vi "WILT Station Controller.vi"(0 "Station Number":u32, 1 "GUI Aisle in":T9[](array[typedef]) {"Night Cycle Count" format="%04d"; "Day Cycle Count" format="%04d"}, 3 "Drying Time (Min)":dbl[](array[numeric]), 4 "Current Threshold":dbl=1.0 format="%#_13g", 5 "Station Test State In":T7, 7 "Error In":errorcluster, 8 "Aisle Location Index":i32, 9 "Cool Down Period (seconds)":dbl[](array[numeric]), 10 "Disable Flood Check":bool, 11 "Delay After Cutout (sec)":dbl=5.0 format="%#_13g", 12 "Previous Run Statistics":T2[](array[typedef]), 13 "Send Restart Every? (Sec)":dbl=7.0 format="%#_13g", 14 "Agilent Valve and Switch Locations":T3[](array[typedef])=[{"Channel"="301", "Station"="1", "Label"="Water Valve", "Agilent Station"="2", "Data"=0.0}, {"Channel"="302", "Station"="2", "Label"="Water Valve", "Agilent Station"="2", "Data"=0.0}, {"Channel"="303", "Station"="3", "Label"="Water Valve", "Agilent Station"="2", "Data"=0.0}, {"Channel"="304", "Station"="4", "Label"="Water Valve", "Agilent Station"="2", "Data"=0.0}, {"Channel"="305", "Station"="5", "Label"="Water Valve", "Agilent Station"="2", "Data"=0.0}, {"Channel"="306", "Station"="6", "Label"="Water Valve", "Agilent Station"="2", "Data"=0.0}, {"Channel"="307", "Station"="7", "Label"="Water Valve", "Agilent Station"="2", "Data"=0.0}, {"Channel"="308", "Station"="8", "Label"="Water Valve", "Agilent Station"="2", "Data"=0.0}, {"Channel"="309", "Station"="9", "Label"="Water Valve", "Agilent Station"="2", "Data"=0.0}, {"Channel"="310", "Station"="10", "Label"="Water Valve", "Agilent Station"="2", "Data"=0.0}, {"Channel"="311", "Station"="11", "Label"="Water Valve", "Agilent Station"="2", "Data"=0.0}, {"Channel"="312", "Station"="12", "Label"="Water Valve", "Agilent Station"="2", "Data"=0.0}, {"Channel"="313", "Station"="13", "Label"="Water Valve", "Agilent Station"="2", "Data"=0.0}, {"Channel"="314", "Station"="14", "Label"="Water Valve", "Agilent Station"="2", "Data"=0.0}, {"Channel"="315", "Station"="15", "Label"="Water Valve", "Agilent Station"="2", "Data"=0.0}, {"Channel"="316", "Station"="16", "Label"="Water Valve", "Agilent Station"="2", "Data"=0.0}, {"Channel"="317", "Station"="17", "Label"="Water Valve", "Agilent Station"="2", "Data"=0.0}, {"Channel"="318", "Station"="18", "Label"="Water Valve", "Agilent Station"="2", "Data"=0.0}, {"Channel"="319", "Station"="19", "Label"="Water Valve", "Agilent Station"="2", "Data"=0.0}, {"Channel"="320", "Station"="20", "Label"="Water Valve", "Agilent Station"="2", "Data"=0.0}, {"Channel"="101", "Station"="21", "Label"="Water Valve", "Agilent Station"="3", "Data"=0.0}, {"Channel"="102", "Station"="22", "Label"="Water Valve", "Agilent Station"="3", "Data"=0.0}, {"Channel"="103", "Station"="23", "Label"="Water Valve", "Agilent Station"="3", "Data"=0.0}, {"Channel"="104", "Station"="24", "Label"="Water Valve", "Agilent Station"="3", "Data"=0.0}, {"Channel"="105", "Station"="25", "Label"="Water Valve", "Agilent Station"="3", "Data"=0.0}, {"Channel"="106", "Station"="26", "Label"="Water Valve", "Agilent Station"="3", "Data"=0.0}, {"Channel"="107", "Station"="27", "Label"="Water Valve", "Agilent Station"="3", "Data"=0.0}, {"Channel"="108", "Station"="28", "Label"="Water Valve", "Agilent Station"="3", "Data"=0.0}, {"Channel"="109", "Station"="29", "Label"="Water Valve", "Agilent Station"="3", "Data"=0.0}, {"Channel"="110", "Station"="30", "Label"="Water Valve", "Agilent Station"="3", "Data"=0.0}, {"Channel"="111", "Station"="31", "Label"="Water Valve", "Agilent Station"="3", "Data"=0.0}, {"Channel"="112", "Station"="32", "Label"="Water Valve", "Agilent Station"="3", "Data"=0.0}, {"Channel"="101", "Station"="33", "Label"="Water Valve", "Agilent Station"="5", "Data"=0.0}, {"Channel"="102", "Station"="34", "Label"="Water Valve", "Agilent Station"="5", "Data"=0.0}, {"Channel"="103", "Station"="35", "Label"="Water Valve", "Agilent Station"="5", "Data"=0.0}, {"Channel"="104", "Station"="36", "Label"="Water Valve", "Agilent Station"="5", "Data"=0.0}, {"Channel"="105", "Station"="37", "Label"="Water Valve", "Agilent Station"="5", "Data"=0.0}, {"Channel"="106", "Station"="38", "Label"="Water Valve", "Agilent Station"="5", "Data"=0.0}, {"Channel"="107", "Station"="39", "Label"="Water Valve", "Agilent Station"="5", "Data"=0.0}, {"Channel"="108", "Station"="40", "Label"="Water Valve", "Agilent Station"="5", "Data"=0.0}, {"Channel"="109", "Station"="41", "Label"="Water Valve", "Agilent Station"="5", "Data"=0.0}, {"Channel"="110", "Station"="42", "Label"="Water Valve", "Agilent Station"="5", "Data"=0.0}, {"Channel"="111", "Station"="43", "Label"="Water Valve", "Agilent Station"="5", "Data"=0.0}, {"Channel"="112", "Station"="44", "Label"="Water Valve", "Agilent Station"="5", "Data"=0.0}, {"Channel"="113", "Station"="45", "Label"="Water Valve", "Agilent Station"="5", "Data"=0.0}, {"Channel"="114", "Station"="46", "Label"="Water Valve", "Agilent Station"="5", "Data"=0.0}, {"Channel"="115", "Station"="47", "Label"="Water Valve", "Agilent Station"="5", "Data"=0.0}, {"Channel"="116", "Station"="48", "Label"="Water Valve", "Agilent Station"="5", "Data"=0.0}, {"Channel"="117", "Station"="49", "Label"="Water Valve", "Agilent Station"="5", "Data"=0.0}, {"Channel"="118", "Station"="50", "Label"="Water Valve", "Agilent Station"="5", "Data"=0.0}, {"Channel"="119", "Station"="51", "Label"="Water Valve", "Agilent Station"="5", "Data"=0.0}, {"Channel"="120", "Station"="52", "Label"="Water Valve", "Agilent Station"="5", "Data"=0.0}, {"Channel"="201", "Station"="53", "Label"="Water Valve", "Agilent Station"="5", "Data"=0.0}, {"Channel"="202", "Station"="54", "Label"="Water Valve", "Agilent Station"="5", "Data"=0.0}, {"Channel"="203", "Station"="55", "Label"="Water Valve", "Agilent Station"="5", "Data"=0.0}, {"Channel"="204", "Station"="56", "Label"="Water Valve", "Agilent Station"="5", "Data"=0.0}, {"Channel"="301", "Station"="21", "Label"="Start Button", "Agilent Station"="5", "Data"=0.0}, {"Channel"="302", "Station"="22", "Label"="Start Button", "Agilent Station"="5", "Data"=0.0}, {"Channel"="303", "Station"="23", "Label"="Start Button", "Agilent Station"="5", "Data"=0.0}, {"Channel"="304", "Station"="24", "Label"="Start Button", "Agilent Station"="5", "Data"=0.0}, {"Channel"="305", "Station"="25", "Label"="Start Button", "Agilent Station"="5", "Data"=0.0}, {"Channel"="306", "Station"="26", "Label"="Start Button", "Agilent Station"="5", "Data"=0.0}, {"Channel"="307", "Station"="27", "Label"="Start Button", "Agilent Station"="5", "Data"=0.0}, {"Channel"="308", "Station"="28", "Label"="Start Button", "Agilent Station"="5", "Data"=0.0}, {"Channel"="309", "Station"="29", "Label"="Start Button", "Agilent Station"="5", "Data"=0.0}, {"Channel"="310", "Station"="30", "Label"="Start Button", "Agilent Station"="5", "Data"=0.0}, {"Channel"="311", "Station"="31", "Label"="Start Button", "Agilent Station"="5", "Data"=0.0}, {"Channel"="312", "Station"="32", "Label"="Start Button", "Agilent Station"="5", "Data"=0.0}, {"Channel"="101", "Station"="33", "Label"="Start Button", "Agilent Station"="7", "Data"=0.0}, {"Channel"="102", "Station"="34", "Label"="Start Button", "Agilent Station"="7", "Data"=0.0}, {"Channel"="103", "Station"="35", "Label"="Start Button", "Agilent Station"="7", "Data"=0.0}, {"Channel"="104", "Station"="36", "Label"="Start Button", "Agilent Station"="7", "Data"=0.0}, {"Channel"="105", "Station"="37", "Label"="Start Button", "Agilent Station"="7", "Data"=0.0}, {"Channel"="106", "Station"="38", "Label"="Start Button", "Agilent Station"="7", "Data"=0.0}, {"Channel"="107", "Station"="39", "Label"="Start Button", "Agilent Station"="7", "Data"=0.0}, {"Channel"="108", "Station"="40", "Label"="Start Button", "Agilent Station"="7", "Data"=0.0}, {"Channel"="109", "Station"="41", "Label"="Start Button", "Agilent Station"="7", "Data"=0.0}, {"Channel"="110", "Station"="42", "Label"="Start Button", "Agilent Station"="7", "Data"=0.0}, {"Channel"="111", "Station"="43", "Label"="Start Button", "Agilent Station"="7", "Data"=0.0}, {"Channel"="112", "Station"="44", "Label"="Start Button", "Agilent Station"="7", "Data"=0.0}, {"Channel"="113", "Station"="45", "Label"="Start Button", "Agilent Station"="7", "Data"=0.0}, {"Channel"="114", "Station"="46", "Label"="Start Button", "Agilent Station"="7", "Data"=0.0}, {"Channel"="115", "Station"="47", "Label"="Start Button", "Agilent Station"="7", "Data"=0.0}, {"Channel"="116", "Station"="48", "Label"="Start Button", "Agilent Station"="7", "Data"=0.0}, {"Channel"="117", "Station"="49", "Label"="Start Button", "Agilent Station"="7", "Data"=0.0}, {"Channel"="118", "Station"="50", "Label"="Start Button", "Agilent Station"="7", "Data"=0.0}, {"Channel"="119", "Station"="51", "Label"="Start Button", "Agilent Station"="7", "Data"=0.0}, {"Channel"="120", "Station"="52", "Label"="Start Button", "Agilent Station"="7", "Data"=0.0}, {"Channel"="201", "Station"="53", "Label"="Start Button", "Agilent Station"="7", "Data"=0.0}, {"Channel"="202", "Station"="54", "Label"="Start Button", "Agilent Station"="7", "Data"=0.0}, {"Channel"="203", "Station"="55", "Label"="Start Button", "Agilent Station"="7", "Data"=0.0}, {"Channel"="204", "Station"="56", "Label"="Start Button", "Agilent Station"="7", "Data"=0.0}], 15 "Injection Times":T4, 16 "Enable Start Retry":bool[](array[boolean]), 17 "Day/Night Cycle":T6, 19 "Final Start Presses":i32=2, 25 "Semaphore":T1[](array[typedef])) -> (20 "GUI Aisle 1":T9[](array[typedef]) {"Night Cycle Count" format="%04d"; "Day Cycle Count" format="%04d"}, 21 "Test Station Out":T7, 23 "Resending Sending Command":bool, 24 "Enable Start Retry Out":bool[](array[boolean]), 27 "Error Out":errorcluster)   [LabVIEW 2016]
uses:
  Type Definitions/WILT Dryer.ctl
  Type Definitions/WILT Dryer Details.ctl
  Type Definitions/WILT Agilent Channel Definition.ctl
  Type Definitions/WILT DAQ Data.ctl
  Type Definitions/WILT Station Test State Cluster.ctl
  Type Definitions/WILT Dryer Test State.ctl
  Type Definitions/WILT Day Night Cycle Enum.ctl
  Type Definitions/WILT Injection Times.ctl
  Type Definitions/WILT Water Injection Control.ctl
  Type Definitions/WILT Summary Data.ctl
  Type Definitions/WILT Water Valve Control.ctl
  Type Definitions/WILT Room Location.ctl
panel:
  out "56":dbl
  out "55":dbl
  out "54":dbl
  out "53":dbl
  out "52":dbl
  out "51":dbl
  out "50":dbl
  out "49":dbl
  out "48":dbl
  out "47":dbl
  out "46":dbl
  out "45":dbl
  out "44":dbl
  out "43":dbl
  out "42":dbl
  out "41":dbl
  out "40":dbl
  out "39":dbl
  out "38":dbl
  out "37":dbl
  out "36":dbl
  out "35":dbl
  out "34":dbl
  out "33":dbl
  out "32":dbl
  out "31":dbl
  out "30":dbl
  out "29":dbl
  out "28":dbl
  out "27":dbl
  out "26":dbl
  out "25":dbl
  out "24":dbl
  out "23":dbl
  out "22":dbl
  out "21":dbl
  out "20":dbl
  out "19":dbl
  out "18":dbl
  out "17":dbl
  out "16":dbl
  out "15":dbl
  out "14":dbl
  out "13":dbl
  out "12":dbl
  out "11":dbl
  out "10":dbl
  out "9":dbl
  out "8":dbl
  out "7":dbl
  out "6":dbl
  out "5":dbl
  out "4":dbl
  out "3":dbl
  out "2":dbl
  out "1":dbl
  # "Individual Station Timers"
  # "Day"
  # "Night"
  # "Day"
  # "Night"
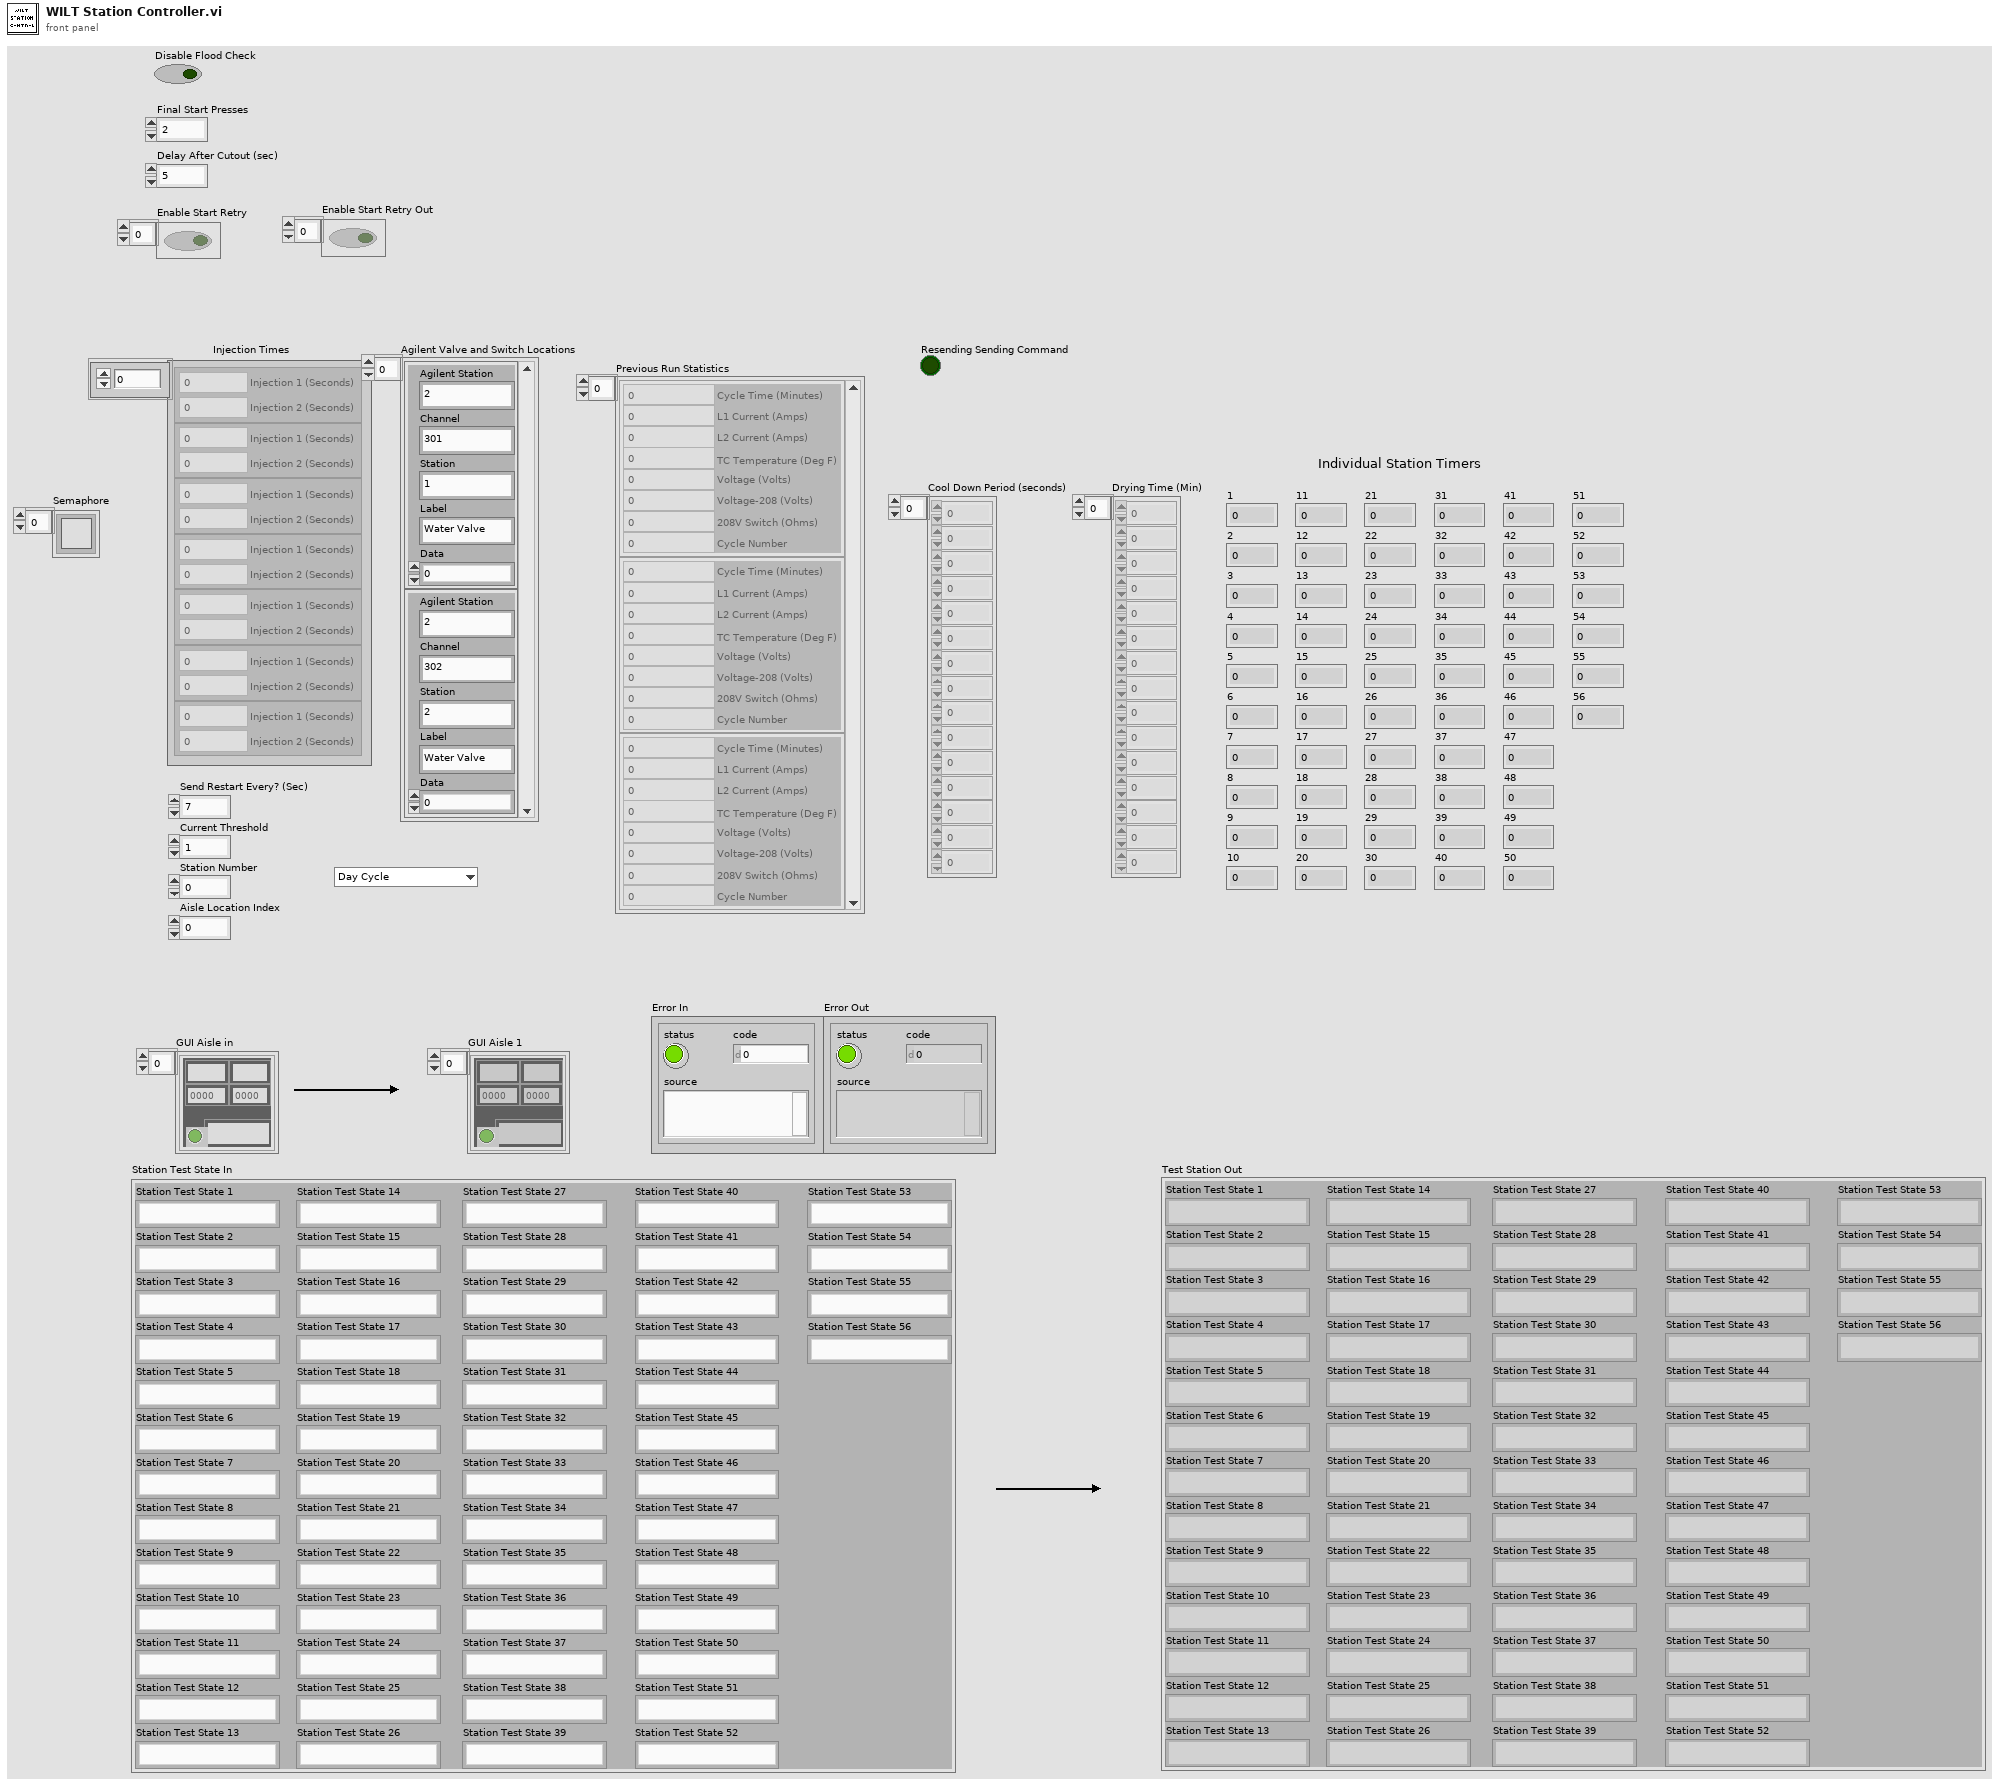
[diagram p1: front panel]
types:
  T1 = typedef "Semaphore RefNum" = refnum<k1>
  T2 = typedef "WILT Summary Data.ctl" = cluster{"Cycle Time (Minutes)":dbl, "L1 Current (Amps)":dbl, "L2 Current (Amps)":dbl, "TC Temperature (Deg F)":dbl, "Voltage (Volts)":dbl, "Voltage-208 (Volts)":dbl, "208V Switch (Ohms)":dbl, "Cycle Number":i32}
  T3 = typedef "WILT Agilent Channel Definition.ctl" = cluster{"Channel":string, "Station":string, "Label":string, "Agilent Station":string, "Data":dbl}
  T4 = typedef "WILT Injection Times.ctl" = T5[]
  T5 = typedef "WILT Water Injection Control.ctl" = cluster{"Injection 1 (Seconds)":dbl, "Injection 2 (Seconds)":dbl}
  T6 = typedef "WILT Day Night Cycle Enum.ctl" = enum16{"Day Cycle", "Night Cycle", "Day Cycle (No Water)"}
  T7 = typedef "WILT Station Test State Cluster.ctl" = cluster{"Station Test State 1":T8, "Station Test State 2":T8, "Station Test State 3":T8, "Station Test State 4":T8, "Station Test State 5":T8, "Station Test State 6":T8, "Station Test State 7":T8, "Station Test State 8":T8, "Station Test State 9":T8, "Station Test State 10":T8, "Station Test State 11":T8, "Station Test State 12":T8, "Station Test State 13":T8, "Station Test State 14":T8, "Station Test State 15":T8, "Station Test State 16":T8, "Station Test State 17":T8, "Station Test State 18":T8, "Station Test State 19":T8, "Station Test State 20":T8, "Station Test State 21":T8, "Station Test State 22":T8, "Station Test State 23":T8, "Station Test State 24":T8, "Station Test State 25":T8, "Station Test State 26":T8, "Station Test State 27":T8, "Station Test State 28":T8, "Station Test State 29":T8, "Station Test State 30":T8, "Station Test State 31":T8, "Station Test State 32":T8, "Station Test State 33":T8, "Station Test State 34":T8, "Station Test State 35":T8, "Station Test State 36":T8, "Station Test State 37":T8, "Station Test State 38":T8, "Station Test State 39":T8, "Station Test State 40":T8, "Station Test State 41":T8, "Station Test State 42":T8, "Station Test State 43":T8, "Station Test State 44":T8, "Station Test State 45":T8, "Station Test State 46":T8, "Station Test State 47":T8, "Station Test State 48":T8, "Station Test State 49":T8, "Station Test State 50":T8, "Station Test State 51":T8, "Station Test State 52":T8, "Station Test State 53":T8, "Station Test State 54":T8, "Station Test State 55":T8, "Station Test State 56":T8}
  T8 = typedef "WILT Dryer Test State.ctl" = enum16{"No Serial Number", "Waiting for Dryer To Start", "Drying Clothes", "Water Injection 1 (On)", "Water Injection 1 Timer", "Water Injection 1 (Off)", "Pause Dryer", "Sending Start Stop CMD", "Pause Dryer 2", "Sending Start Stop CMD 2", "Drying Clothes 2", "Water Injection 2 (On)", "Water Injection 2 Timer", "Water Injection 2 (Off)", "Drying Clothes 3", "Cooling Down", "Sending Start Stop CMD 3", "Increment Cycle"}
  T9 = typedef "WILT Dryer.ctl" = cluster{"Lab ID":string, "Day Cycle Count":i32, "Station Label":string, "Dryer Details":T10, "Status Color":u32, "Invisible Button":bool, "Night Cycle Count":i32, "Station Index":i32, "Cycle Index":string, "Audit Alert":bool, "Agilent Channel Definition":T3, "DAQ Data":T11}
  T10 = typedef "WILT Dryer Details.ctl" = cluster{"Station":string, "Lab ID":string, "TR Number":string}
  T11 = typedef "WILT DAQ Data.ctl" = cluster{"L1 Current":dbl, "L2 Current":dbl, "Temperature  Deg F (TC)":dbl, "Volts":dbl, "Volts (208)":dbl, "SW (208)":dbl}
  T12 = typedef "WILT Room Location.ctl" = enum16{"Big Room", "Remote Stations"}
  T13 = typedef "WILT Water Valve Control.ctl" = enum16{"Turn Valve ON (Injection 1)", "Turn Valve OFF (Injection 1)", "Turn Valve ON (Injection 2)", "Turn Valve OFF (Injection 2)"}
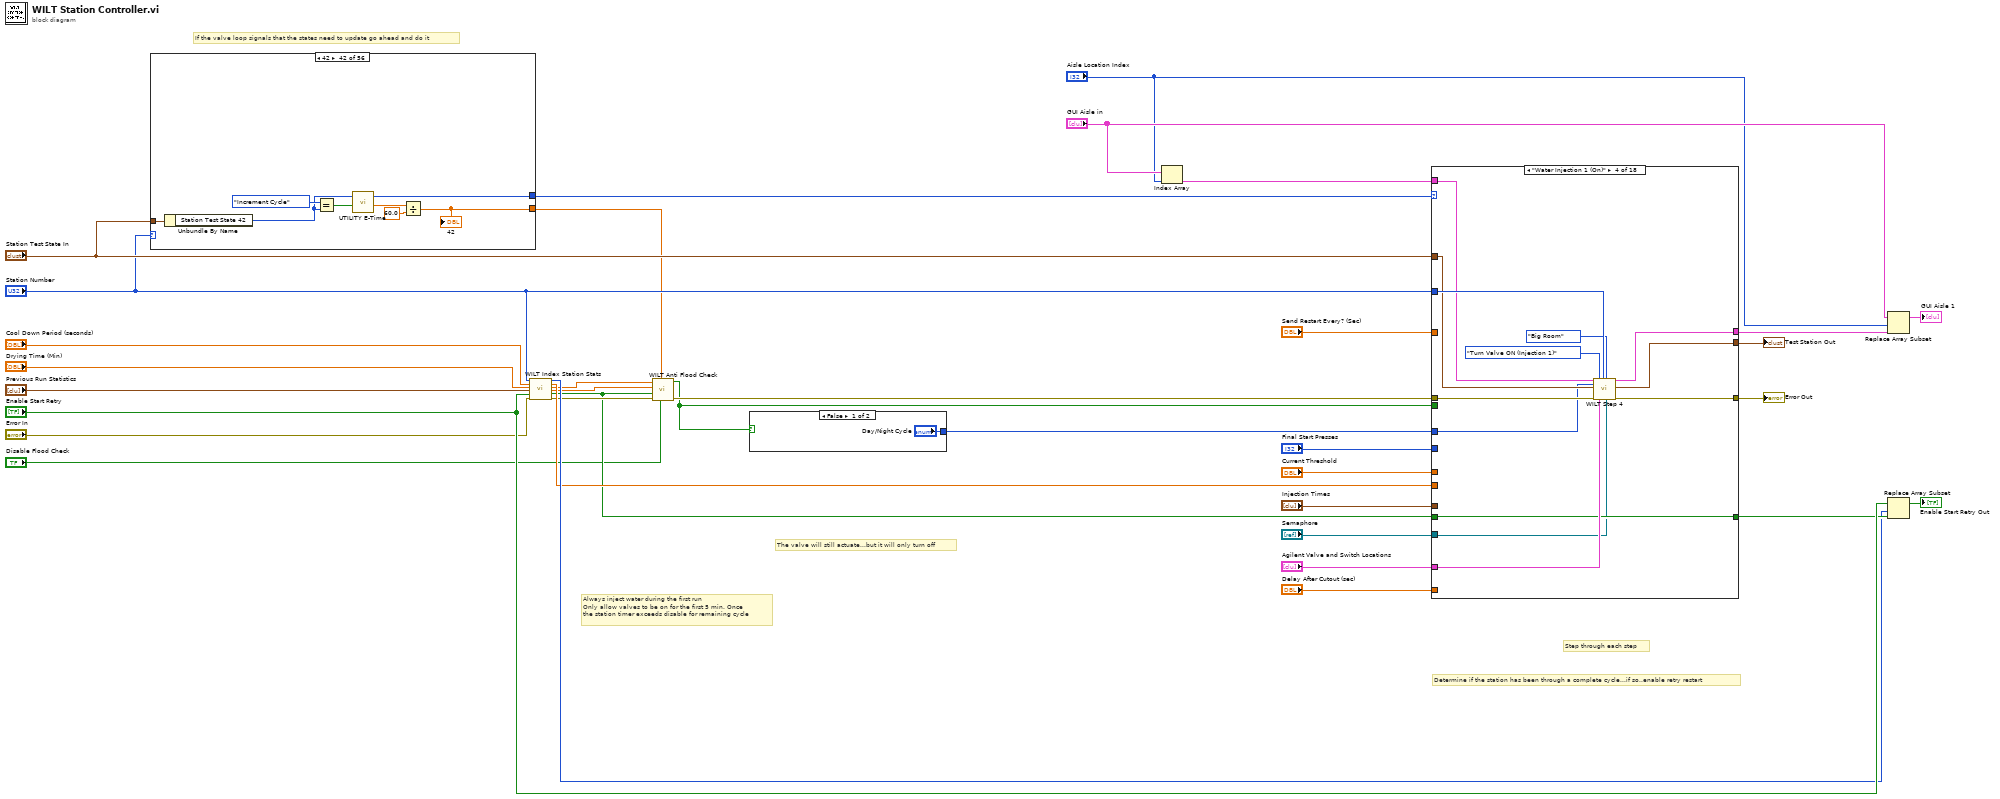
[diagram p0: block diagram]
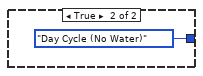
[diagram p2: hidden frame]
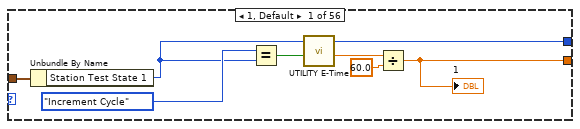
[diagram p3: hidden frame]
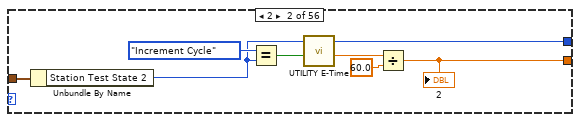
[diagram p4: hidden frame]
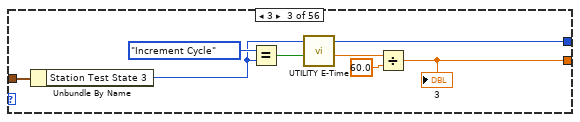
[diagram p5: hidden frame]
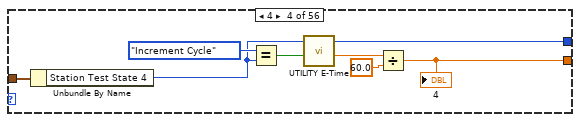
[diagram p6: hidden frame]
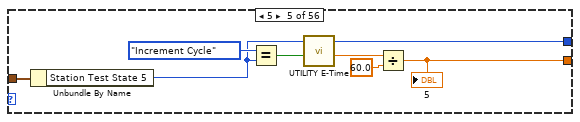
[diagram p7: hidden frame]
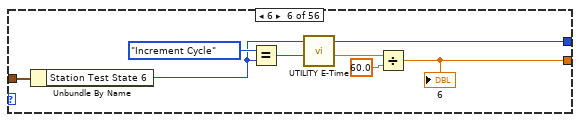
[diagram p8: hidden frame]
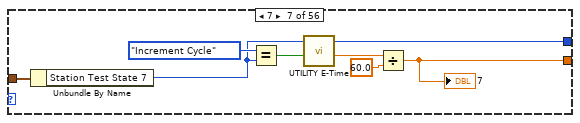
[diagram p9: hidden frame]
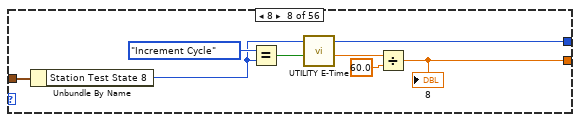
[diagram p10: hidden frame]
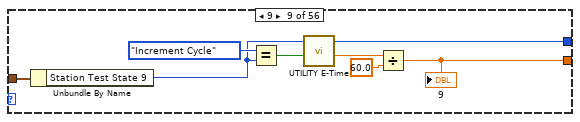
[diagram p11: hidden frame]
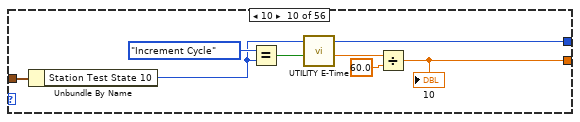
[diagram p12: hidden frame]
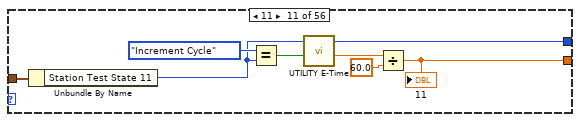
[diagram p13: hidden frame]
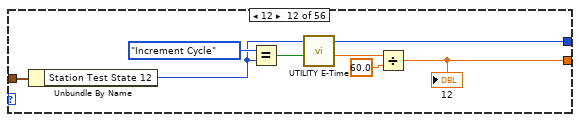
[diagram p14: hidden frame]
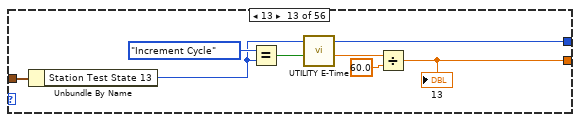
[diagram p15: hidden frame]
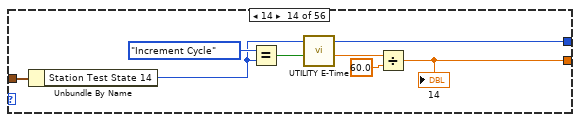
[diagram p16: hidden frame]
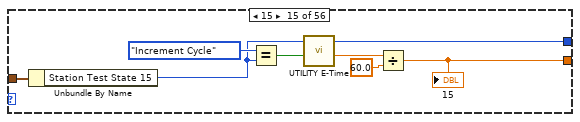
[diagram p17: hidden frame]
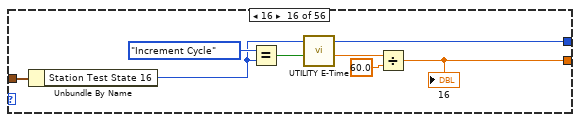
[diagram p18: hidden frame]
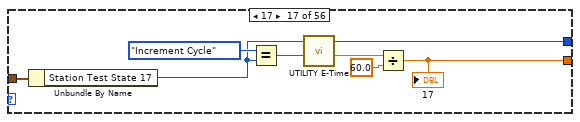
[diagram p19: hidden frame]
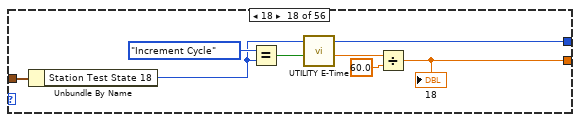
[diagram p20: hidden frame]
diagram:
  # "The valve will still actuate...but it will only turn off"
  # "Always inject water during the first run\nOnly allow valves to be on for the first 5 min. Once\nthe station timer exceeds disable for remaining cycle"
  # "Determine if the station has been through a complete cycle...if so..enable retry restart"
  # "Step through each step"
  # "If the valve loop signals that the states need to update go ahead and do it"
  n1 = case shown="42" "Station Number" {
    tunnel: "Station Test State In" -> [w42 w49 w56 w63 w70 w77 w84 w91 w98 w105 w112 w119 w126 w133 w140 w147 w154 w161 w168 w175 w182 w189 w196 w203 w210 w217 w224 w231 w238 w245 w252 w259 w266 w273 w280 w287 w294 w301 w308 w315 w322 w329 w336 w343 w350 w357 w364 w371 w378 w385 w392 w399 w406 w413 w420 w427]
    tunnel: [w37 w44 w51 w58 w65 w72 w79 w86 w93 w100 w107 w114 w121 w128 w135 w142 w149 w156 w163 w170 w181 w184 w191 w198 w205 w212 w219 w226 w233 w240 w247 w254 w261 w268 w275 w282 w289 w296 w303 w310 w317 w324 w331 w338 w345 w352 w359 w366 w373 w380 w387 w394 w401 w408 w415 w422] -> w31
    tunnel: [w36 w43 w50 w57 w64 w71 w78 w85 w92 w99 w106 w113 w120 w127 w134 w141 w148 w155 w162 w169 w176 w183 w190 w197 w204 w211 w218 w225 w232 w239 w246 w253 w260 w267 w274 w281 w288 w295 w302 w309 w316 w323 w330 w337 w344 w351 w358 w365 w372 w379 w386 w393 w400 w407 w414 w421] -> w5
    frame 1, Default {
      n2 = Unbundle By Name(w42) -> ("Station Test State 1"=w37:T8)
      n3 = Equal?(x=WILT_Dryer_Test_State."Increment Cycle", y=w37) -> (x = y?=w39:bool)
      n4 = call "UTILITY E-Time.vi"("Reset"=w39) -> ("Elapsed Time (sec)"=w38:dbl)  [unwired: 8 in, 2 out]
      n5 = Divide(x=w38, y=60.0) -> (x/y=w36:dbl)
      "1" <- w36
    }
    frame 2 {
      n6 = Unbundle By Name(w49) -> ("Station Test State 2"=w44:T8)
      n7 = Equal?(x=WILT_Dryer_Test_State."Increment Cycle", y=w44) -> (x = y?=w46:bool)
      n8 = call "UTILITY E-Time.vi"("Reset"=w46) -> ("Elapsed Time (sec)"=w45:dbl)  [unwired: 8 in, 2 out]
      n9 = Divide(x=w45, y=60.0) -> (x/y=w43:dbl)
      "2" <- w43
    }
    frame 3 {
      n10 = Unbundle By Name(w56) -> ("Station Test State 3"=w51:T8)
      n11 = Equal?(x=WILT_Dryer_Test_State."Increment Cycle", y=w51) -> (x = y?=w53:bool)
      n12 = call "UTILITY E-Time.vi"("Reset"=w53) -> ("Elapsed Time (sec)"=w52:dbl)  [unwired: 8 in, 2 out]
      n13 = Divide(x=w52, y=60.0) -> (x/y=w50:dbl)
      "3" <- w50
    }
    frame 4 {
      n14 = Unbundle By Name(w63) -> ("Station Test State 4"=w58:T8)
      n15 = Equal?(x=WILT_Dryer_Test_State."Increment Cycle", y=w58) -> (x = y?=w60:bool)
      n16 = call "UTILITY E-Time.vi"("Reset"=w60) -> ("Elapsed Time (sec)"=w59:dbl)  [unwired: 8 in, 2 out]
      n17 = Divide(x=w59, y=60.0) -> (x/y=w57:dbl)
      "4" <- w57
    }
    frame 5 {
      n18 = Unbundle By Name(w70) -> ("Station Test State 5"=w65:T8)
      n19 = Equal?(x=WILT_Dryer_Test_State."Increment Cycle", y=w65) -> (x = y?=w67:bool)
      n20 = call "UTILITY E-Time.vi"("Reset"=w67) -> ("Elapsed Time (sec)"=w66:dbl)  [unwired: 8 in, 2 out]
      n21 = Divide(x=w66, y=60.0) -> (x/y=w64:dbl)
      "5" <- w64
    }
    frame 6 {
      n22 = Unbundle By Name(w77) -> ("Station Test State 6"=w72:T8)
      n23 = Equal?(x=WILT_Dryer_Test_State."Increment Cycle", y=w72) -> (x = y?=w74:bool)
      n24 = call "UTILITY E-Time.vi"("Reset"=w74) -> ("Elapsed Time (sec)"=w73:dbl)  [unwired: 8 in, 2 out]
      n25 = Divide(x=w73, y=60.0) -> (x/y=w71:dbl)
      "6" <- w71
    }
    frame 7 {
      n26 = Unbundle By Name(w84) -> ("Station Test State 7"=w79:T8)
      n27 = Equal?(x=WILT_Dryer_Test_State."Increment Cycle", y=w79) -> (x = y?=w81:bool)
      n28 = call "UTILITY E-Time.vi"("Reset"=w81) -> ("Elapsed Time (sec)"=w80:dbl)  [unwired: 8 in, 2 out]
      n29 = Divide(x=w80, y=60.0) -> (x/y=w78:dbl)
      "7" <- w78
    }
    frame 8 {
      n30 = Unbundle By Name(w91) -> ("Station Test State 8"=w86:T8)
      n31 = Equal?(x=WILT_Dryer_Test_State."Increment Cycle", y=w86) -> (x = y?=w88:bool)
      n32 = call "UTILITY E-Time.vi"("Reset"=w88) -> ("Elapsed Time (sec)"=w87:dbl)  [unwired: 8 in, 2 out]
      n33 = Divide(x=w87, y=60.0) -> (x/y=w85:dbl)
      "8" <- w85
    }
    frame 9 {
      n34 = Unbundle By Name(w98) -> ("Station Test State 9"=w93:T8)
      n35 = Equal?(x=WILT_Dryer_Test_State."Increment Cycle", y=w93) -> (x = y?=w95:bool)
      n36 = call "UTILITY E-Time.vi"("Reset"=w95) -> ("Elapsed Time (sec)"=w94:dbl)  [unwired: 8 in, 2 out]
      n37 = Divide(x=w94, y=60.0) -> (x/y=w92:dbl)
      "9" <- w92
    }
    frame 10 {
      n38 = Unbundle By Name(w105) -> ("Station Test State 10"=w100:T8)
      n39 = Equal?(x=WILT_Dryer_Test_State."Increment Cycle", y=w100) -> (x = y?=w102:bool)
      n40 = call "UTILITY E-Time.vi"("Reset"=w102) -> ("Elapsed Time (sec)"=w101:dbl)  [unwired: 8 in, 2 out]
      n41 = Divide(x=w101, y=60.0) -> (x/y=w99:dbl)
      "10" <- w99
    }
    frame 11 {
      n42 = Unbundle By Name(w112) -> ("Station Test State 11"=w107:T8)
      n43 = Equal?(x=WILT_Dryer_Test_State."Increment Cycle", y=w107) -> (x = y?=w109:bool)
      n44 = call "UTILITY E-Time.vi"("Reset"=w109) -> ("Elapsed Time (sec)"=w108:dbl)  [unwired: 8 in, 2 out]
      n45 = Divide(x=w108, y=60.0) -> (x/y=w106:dbl)
      "11" <- w106
    }
    frame 12 {
      n46 = Unbundle By Name(w119) -> ("Station Test State 12"=w114:T8)
      n47 = Equal?(x=WILT_Dryer_Test_State."Increment Cycle", y=w114) -> (x = y?=w116:bool)
      n48 = call "UTILITY E-Time.vi"("Reset"=w116) -> ("Elapsed Time (sec)"=w115:dbl)  [unwired: 8 in, 2 out]
      n49 = Divide(x=w115, y=60.0) -> (x/y=w113:dbl)
      "12" <- w113
    }
    frame 13 {
      n50 = Unbundle By Name(w126) -> ("Station Test State 13"=w121:T8)
      n51 = Equal?(x=WILT_Dryer_Test_State."Increment Cycle", y=w121) -> (x = y?=w123:bool)
      n52 = call "UTILITY E-Time.vi"("Reset"=w123) -> ("Elapsed Time (sec)"=w122:dbl)  [unwired: 8 in, 2 out]
      n53 = Divide(x=w122, y=60.0) -> (x/y=w120:dbl)
      "13" <- w120
    }
    frame 14 {
      n54 = Unbundle By Name(w133) -> ("Station Test State 14"=w128:T8)
      n55 = Equal?(x=WILT_Dryer_Test_State."Increment Cycle", y=w128) -> (x = y?=w130:bool)
      n56 = call "UTILITY E-Time.vi"("Reset"=w130) -> ("Elapsed Time (sec)"=w129:dbl)  [unwired: 8 in, 2 out]
      n57 = Divide(x=w129, y=60.0) -> (x/y=w127:dbl)
      "14" <- w127
    }
    frame 15 {
      n58 = Unbundle By Name(w140) -> ("Station Test State 15"=w135:T8)
      n59 = Equal?(x=WILT_Dryer_Test_State."Increment Cycle", y=w135) -> (x = y?=w137:bool)
      n60 = call "UTILITY E-Time.vi"("Reset"=w137) -> ("Elapsed Time (sec)"=w136:dbl)  [unwired: 8 in, 2 out]
      n61 = Divide(x=w136, y=60.0) -> (x/y=w134:dbl)
      "15" <- w134
    }
    frame 16 {
      n62 = Unbundle By Name(w147) -> ("Station Test State 16"=w142:T8)
      n63 = Equal?(x=WILT_Dryer_Test_State."Increment Cycle", y=w142) -> (x = y?=w144:bool)
      n64 = call "UTILITY E-Time.vi"("Reset"=w144) -> ("Elapsed Time (sec)"=w143:dbl)  [unwired: 8 in, 2 out]
      n65 = Divide(x=w143, y=60.0) -> (x/y=w141:dbl)
      "16" <- w141
    }
    frame 17 {
      n66 = Unbundle By Name(w154) -> ("Station Test State 17"=w149:T8)
      n67 = Equal?(x=WILT_Dryer_Test_State."Increment Cycle", y=w149) -> (x = y?=w151:bool)
      n68 = call "UTILITY E-Time.vi"("Reset"=w151) -> ("Elapsed Time (sec)"=w150:dbl)  [unwired: 8 in, 2 out]
      n69 = Divide(x=w150, y=60.0) -> (x/y=w148:dbl)
      "17" <- w148
    }
    frame 18 {
      n70 = Unbundle By Name(w161) -> ("Station Test State 18"=w156:T8)
      n71 = Equal?(x=WILT_Dryer_Test_State."Increment Cycle", y=w156) -> (x = y?=w158:bool)
      n72 = call "UTILITY E-Time.vi"("Reset"=w158) -> ("Elapsed Time (sec)"=w157:dbl)  [unwired: 8 in, 2 out]
      n73 = Divide(x=w157, y=60.0) -> (x/y=w155:dbl)
      "18" <- w155
    }
    frame 19 {
      n74 = Unbundle By Name(w168) -> ("Station Test State 19"=w163:T8)
      n75 = Equal?(x=WILT_Dryer_Test_State."Increment Cycle", y=w163) -> (x = y?=w165:bool)
      n76 = call "UTILITY E-Time.vi"("Reset"=w165) -> ("Elapsed Time (sec)"=w164:dbl)  [unwired: 8 in, 2 out]
      n77 = Divide(x=w164, y=60.0) -> (x/y=w162:dbl)
      "19" <- w162
    }
    frame 20 {
      n78 = Unbundle By Name(w175) -> ("Station Test State 20"=w170:T8)
      n79 = Equal?(x=WILT_Dryer_Test_State."Increment Cycle", y=w170) -> (x = y?=w172:bool)
      n80 = call "UTILITY E-Time.vi"("Reset"=w172) -> ("Elapsed Time (sec)"=w171:dbl)  [unwired: 8 in, 2 out]
      n81 = Divide(x=w171, y=60.0) -> (x/y=w169:dbl)
      "20" <- w169
    }
    frame 21 {
      n82 = Unbundle By Name(w182) -> ("Station Test State 21"=w181:T8)
      n83 = Equal?(x=WILT_Dryer_Test_State."Increment Cycle", y=w181) -> (x = y?=w178:bool)
      n84 = call "UTILITY E-Time.vi"("Reset"=w178) -> ("Elapsed Time (sec)"=w177:dbl)  [unwired: 8 in, 2 out]
      n85 = Divide(x=w177, y=60.0) -> (x/y=w176:dbl)
      "21" <- w176
    }
    frame 22 {
      n86 = Unbundle By Name(w189) -> ("Station Test State 22"=w184:T8)
      n87 = Equal?(x=WILT_Dryer_Test_State."Increment Cycle", y=w184) -> (x = y?=w186:bool)
      n88 = call "UTILITY E-Time.vi"("Reset"=w186) -> ("Elapsed Time (sec)"=w185:dbl)  [unwired: 8 in, 2 out]
      n89 = Divide(x=w185, y=60.0) -> (x/y=w183:dbl)
      "22" <- w183
    }
    frame 23 {
      n90 = Unbundle By Name(w196) -> ("Station Test State 23"=w191:T8)
      n91 = Equal?(x=WILT_Dryer_Test_State."Increment Cycle", y=w191) -> (x = y?=w193:bool)
      n92 = call "UTILITY E-Time.vi"("Reset"=w193) -> ("Elapsed Time (sec)"=w192:dbl)  [unwired: 8 in, 2 out]
      n93 = Divide(x=w192, y=60.0) -> (x/y=w190:dbl)
      "23" <- w190
    }
    frame 24 {
      n94 = Unbundle By Name(w203) -> ("Station Test State 24"=w198:T8)
      n95 = Equal?(x=WILT_Dryer_Test_State."Increment Cycle", y=w198) -> (x = y?=w200:bool)
      n96 = call "UTILITY E-Time.vi"("Reset"=w200) -> ("Elapsed Time (sec)"=w199:dbl)  [unwired: 8 in, 2 out]
      n97 = Divide(x=w199, y=60.0) -> (x/y=w197:dbl)
      "24" <- w197
    }
    frame 25 {
      n98 = Unbundle By Name(w210) -> ("Station Test State 25"=w205:T8)
      n99 = Equal?(x=WILT_Dryer_Test_State."Increment Cycle", y=w205) -> (x = y?=w207:bool)
      n100 = call "UTILITY E-Time.vi"("Reset"=w207) -> ("Elapsed Time (sec)"=w206:dbl)  [unwired: 8 in, 2 out]
      n101 = Divide(x=w206, y=60.0) -> (x/y=w204:dbl)
      "25" <- w204
    }
    frame 26 {
      n102 = Unbundle By Name(w217) -> ("Station Test State 26"=w212:T8)
      n103 = Equal?(x=WILT_Dryer_Test_State."Increment Cycle", y=w212) -> (x = y?=w214:bool)
      n104 = call "UTILITY E-Time.vi"("Reset"=w214) -> ("Elapsed Time (sec)"=w213:dbl)  [unwired: 8 in, 2 out]
      n105 = Divide(x=w213, y=60.0) -> (x/y=w211:dbl)
      "26" <- w211
    }
    frame 27 {
      n106 = Unbundle By Name(w224) -> ("Station Test State 27"=w219:T8)
      n107 = Equal?(x=WILT_Dryer_Test_State."Increment Cycle", y=w219) -> (x = y?=w221:bool)
      n108 = call "UTILITY E-Time.vi"("Reset"=w221) -> ("Elapsed Time (sec)"=w220:dbl)  [unwired: 8 in, 2 out]
      n109 = Divide(x=w220, y=60.0) -> (x/y=w218:dbl)
      "27" <- w218
    }
    frame 28 {
      n110 = Unbundle By Name(w231) -> ("Station Test State 28"=w226:T8)
      n111 = Equal?(x=WILT_Dryer_Test_State."Increment Cycle", y=w226) -> (x = y?=w228:bool)
      n112 = call "UTILITY E-Time.vi"("Reset"=w228) -> ("Elapsed Time (sec)"=w227:dbl)  [unwired: 8 in, 2 out]
      n113 = Divide(x=w227, y=60.0) -> (x/y=w225:dbl)
      "28" <- w225
    }
    frame 29 {
      n114 = Unbundle By Name(w238) -> ("Station Test State 29"=w233:T8)
      n115 = Equal?(x=WILT_Dryer_Test_State."Increment Cycle", y=w233) -> (x = y?=w235:bool)
      n116 = call "UTILITY E-Time.vi"("Reset"=w235) -> ("Elapsed Time (sec)"=w234:dbl)  [unwired: 8 in, 2 out]
      n117 = Divide(x=w234, y=60.0) -> (x/y=w232:dbl)
      "29" <- w232
    }
    frame 30 {
      n118 = Unbundle By Name(w245) -> ("Station Test State 30"=w240:T8)
      n119 = Equal?(x=WILT_Dryer_Test_State."Increment Cycle", y=w240) -> (x = y?=w242:bool)
      n120 = call "UTILITY E-Time.vi"("Reset"=w242) -> ("Elapsed Time (sec)"=w241:dbl)  [unwired: 8 in, 2 out]
      n121 = Divide(x=w241, y=60.0) -> (x/y=w239:dbl)
      "30" <- w239
    }
    frame 31 {
      n122 = Unbundle By Name(w252) -> ("Station Test State 31"=w247:T8)
      n123 = Equal?(x=WILT_Dryer_Test_State."Increment Cycle", y=w247) -> (x = y?=w249:bool)
      n124 = call "UTILITY E-Time.vi"("Reset"=w249) -> ("Elapsed Time (sec)"=w248:dbl)  [unwired: 8 in, 2 out]
      n125 = Divide(x=w248, y=60.0) -> (x/y=w246:dbl)
      "31" <- w246
    }
    frame 32 {
      n126 = Unbundle By Name(w259) -> ("Station Test State 32"=w254:T8)
      n127 = Equal?(x=WILT_Dryer_Test_State."Increment Cycle", y=w254) -> (x = y?=w256:bool)
      n128 = call "UTILITY E-Time.vi"("Reset"=w256) -> ("Elapsed Time (sec)"=w255:dbl)  [unwired: 8 in, 2 out]
      n129 = Divide(x=w255, y=60.0) -> (x/y=w253:dbl)
      "32" <- w253
    }
    frame 33 {
      n130 = Unbundle By Name(w266) -> ("Station Test State 33"=w261:T8)
      n131 = Equal?(x=WILT_Dryer_Test_State."Increment Cycle", y=w261) -> (x = y?=w263:bool)
      n132 = call "UTILITY E-Time.vi"("Reset"=w263) -> ("Elapsed Time (sec)"=w262:dbl)  [unwired: 8 in, 2 out]
      n133 = Divide(x=w262, y=60.0) -> (x/y=w260:dbl)
      "33" <- w260
    }
    frame 34 {
      n134 = Unbundle By Name(w273) -> ("Station Test State 34"=w268:T8)
      n135 = Equal?(x=WILT_Dryer_Test_State."Increment Cycle", y=w268) -> (x = y?=w270:bool)
      n136 = call "UTILITY E-Time.vi"("Reset"=w270) -> ("Elapsed Time (sec)"=w269:dbl)  [unwired: 8 in, 2 out]
      n137 = Divide(x=w269, y=60.0) -> (x/y=w267:dbl)
      "34" <- w267
    }
    frame 35 {
      n138 = Unbundle By Name(w280) -> ("Station Test State 35"=w275:T8)
      n139 = Equal?(x=WILT_Dryer_Test_State."Increment Cycle", y=w275) -> (x = y?=w277:bool)
      n140 = call "UTILITY E-Time.vi"("Reset"=w277) -> ("Elapsed Time (sec)"=w276:dbl)  [unwired: 8 in, 2 out]
      n141 = Divide(x=w276, y=60.0) -> (x/y=w274:dbl)
      "35" <- w274
    }
    frame 36 {
      n142 = Unbundle By Name(w287) -> ("Station Test State 36"=w282:T8)
      n143 = Equal?(x=WILT_Dryer_Test_State."Increment Cycle", y=w282) -> (x = y?=w284:bool)
      n144 = call "UTILITY E-Time.vi"("Reset"=w284) -> ("Elapsed Time (sec)"=w283:dbl)  [unwired: 8 in, 2 out]
      n145 = Divide(x=w283, y=60.0) -> (x/y=w281:dbl)
      "36" <- w281
    }
    frame 37 {
      n146 = Unbundle By Name(w294) -> ("Station Test State 37"=w289:T8)
      n147 = Equal?(x=WILT_Dryer_Test_State."Increment Cycle", y=w289) -> (x = y?=w291:bool)
      n148 = call "UTILITY E-Time.vi"("Reset"=w291) -> ("Elapsed Time (sec)"=w290:dbl)  [unwired: 8 in, 2 out]
      n149 = Divide(x=w290, y=60.0) -> (x/y=w288:dbl)
      "37" <- w288
    }
    frame 38 {
      n150 = Unbundle By Name(w301) -> ("Station Test State 38"=w296:T8)
      n151 = Equal?(x=WILT_Dryer_Test_State."Increment Cycle", y=w296) -> (x = y?=w298:bool)
      n152 = call "UTILITY E-Time.vi"("Reset"=w298) -> ("Elapsed Time (sec)"=w297:dbl)  [unwired: 8 in, 2 out]
      n153 = Divide(x=w297, y=60.0) -> (x/y=w295:dbl)
      "38" <- w295
    }
    frame 39 {
      n154 = Unbundle By Name(w308) -> ("Station Test State 39"=w303:T8)
      n155 = Equal?(x=WILT_Dryer_Test_State."Increment Cycle", y=w303) -> (x = y?=w305:bool)
      n156 = call "UTILITY E-Time.vi"("Reset"=w305) -> ("Elapsed Time (sec)"=w304:dbl)  [unwired: 8 in, 2 out]
      n157 = Divide(x=w304, y=60.0) -> (x/y=w302:dbl)
      "39" <- w302
    }
    frame 40 {
      n158 = Unbundle By Name(w315) -> ("Station Test State 40"=w310:T8)
      n159 = Equal?(x=WILT_Dryer_Test_State."Increment Cycle", y=w310) -> (x = y?=w312:bool)
      n160 = call "UTILITY E-Time.vi"("Reset"=w312) -> ("Elapsed Time (sec)"=w311:dbl)  [unwired: 8 in, 2 out]
      n161 = Divide(x=w311, y=60.0) -> (x/y=w309:dbl)
      "40" <- w309
    }
    frame 41 {
      n162 = Unbundle By Name(w322) -> ("Station Test State 41"=w317:T8)
      n163 = Equal?(x=WILT_Dryer_Test_State."Increment Cycle", y=w317) -> (x = y?=w319:bool)
      n164 = call "UTILITY E-Time.vi"("Reset"=w319) -> ("Elapsed Time (sec)"=w318:dbl)  [unwired: 8 in, 2 out]
      n165 = Divide(x=w318, y=60.0) -> (x/y=w316:dbl)
      "41" <- w316
    }
    frame 42 {
      n166 = Unbundle By Name(w329) -> ("Station Test State 42"=w324:T8)
      n167 = Equal?(x=WILT_Dryer_Test_State."Increment Cycle", y=w324) -> (x = y?=w326:bool)
      n168 = call "UTILITY E-Time.vi"("Reset"=w326) -> ("Elapsed Time (sec)"=w325:dbl)  [unwired: 8 in, 2 out]
      n169 = Divide(x=w325, y=60.0) -> (x/y=w323:dbl)
      "42" <- w323
    }
    frame 43 {
      n170 = Unbundle By Name(w336) -> ("Station Test State 43"=w331:T8)
      n171 = Equal?(x=WILT_Dryer_Test_State."Increment Cycle", y=w331) -> (x = y?=w333:bool)
      n172 = call "UTILITY E-Time.vi"("Reset"=w333) -> ("Elapsed Time (sec)"=w332:dbl)  [unwired: 8 in, 2 out]
      n173 = Divide(x=w332, y=60.0) -> (x/y=w330:dbl)
      "43" <- w330
    }
    frame 44 {
      n174 = Unbundle By Name(w343) -> ("Station Test State 44"=w338:T8)
      n175 = Equal?(x=WILT_Dryer_Test_State."Increment Cycle", y=w338) -> (x = y?=w340:bool)
      n176 = call "UTILITY E-Time.vi"("Reset"=w340) -> ("Elapsed Time (sec)"=w339:dbl)  [unwired: 8 in, 2 out]
      n177 = Divide(x=w339, y=60.0) -> (x/y=w337:dbl)
      "44" <- w337
    }
    frame 45 {
      n178 = Unbundle By Name(w350) -> ("Station Test State 45"=w345:T8)
      n179 = Equal?(x=WILT_Dryer_Test_State."Increment Cycle", y=w345) -> (x = y?=w347:bool)
      n180 = call "UTILITY E-Time.vi"("Reset"=w347) -> ("Elapsed Time (sec)"=w346:dbl)  [unwired: 8 in, 2 out]
      n181 = Divide(x=w346, y=60.0) -> (x/y=w344:dbl)
      "45" <- w344
    }
    frame 46 {
      n182 = Unbundle By Name(w357) -> ("Station Test State 46"=w352:T8)
      n183 = Equal?(x=WILT_Dryer_Test_State."Increment Cycle", y=w352) -> (x = y?=w354:bool)
      n184 = call "UTILITY E-Time.vi"("Reset"=w354) -> ("Elapsed Time (sec)"=w353:dbl)  [unwired: 8 in, 2 out]
      n185 = Divide(x=w353, y=60.0) -> (x/y=w351:dbl)
      "46" <- w351
    }
    frame 47 {
      n186 = Unbundle By Name(w364) -> ("Station Test State 47"=w359:T8)
      n187 = Equal?(x=WILT_Dryer_Test_State."Increment Cycle", y=w359) -> (x = y?=w361:bool)
      n188 = call "UTILITY E-Time.vi"("Reset"=w361) -> ("Elapsed Time (sec)"=w360:dbl)  [unwired: 8 in, 2 out]
      n189 = Divide(x=w360, y=60.0) -> (x/y=w358:dbl)
      "47" <- w358
    }
    frame 48 {
      n190 = Unbundle By Name(w371) -> ("Station Test State 48"=w366:T8)
      n191 = Equal?(x=WILT_Dryer_Test_State."Increment Cycle", y=w366) -> (x = y?=w368:bool)
      n192 = call "UTILITY E-Time.vi"("Reset"=w368) -> ("Elapsed Time (sec)"=w367:dbl)  [unwired: 8 in, 2 out]
      n193 = Divide(x=w367, y=60.0) -> (x/y=w365:dbl)
      "48" <- w365
    }
    frame 49 {
      n194 = Unbundle By Name(w378) -> ("Station Test State 49"=w373:T8)
      n195 = Equal?(x=WILT_Dryer_Test_State."Increment Cycle", y=w373) -> (x = y?=w375:bool)
      n196 = call "UTILITY E-Time.vi"("Reset"=w375) -> ("Elapsed Time (sec)"=w374:dbl)  [unwired: 8 in, 2 out]
      n197 = Divide(x=w374, y=60.0) -> (x/y=w372:dbl)
      "49" <- w372
    }
    frame 50 {
      n198 = Unbundle By Name(w385) -> ("Station Test State 50"=w380:T8)
      n199 = Equal?(x=WILT_Dryer_Test_State."Increment Cycle", y=w380) -> (x = y?=w382:bool)
      n200 = call "UTILITY E-Time.vi"("Reset"=w382) -> ("Elapsed Time (sec)"=w381:dbl)  [unwired: 8 in, 2 out]
      n201 = Divide(x=w381, y=60.0) -> (x/y=w379:dbl)
      "50" <- w379
    }
    frame 51 {
      n202 = Unbundle By Name(w392) -> ("Station Test State 51"=w387:T8)
      n203 = Equal?(x=WILT_Dryer_Test_State."Increment Cycle", y=w387) -> (x = y?=w389:bool)
      n204 = call "UTILITY E-Time.vi"("Reset"=w389) -> ("Elapsed Time (sec)"=w388:dbl)  [unwired: 8 in, 2 out]
      n205 = Divide(x=w388, y=60.0) -> (x/y=w386:dbl)
      "51" <- w386
    }
    frame 52 {
      n206 = Unbundle By Name(w399) -> ("Station Test State 52"=w394:T8)
      n207 = Equal?(x=WILT_Dryer_Test_State."Increment Cycle", y=w394) -> (x = y?=w396:bool)
      n208 = call "UTILITY E-Time.vi"("Reset"=w396) -> ("Elapsed Time (sec)"=w395:dbl)  [unwired: 8 in, 2 out]
      n209 = Divide(x=w395, y=60.0) -> (x/y=w393:dbl)
      "52" <- w393
    }
    frame 53 {
      n210 = Unbundle By Name(w406) -> ("Station Test State 53"=w401:T8)
      n211 = Equal?(x=WILT_Dryer_Test_State."Increment Cycle", y=w401) -> (x = y?=w403:bool)
      n212 = call "UTILITY E-Time.vi"("Reset"=w403) -> ("Elapsed Time (sec)"=w402:dbl)  [unwired: 8 in, 2 out]
      n213 = Divide(x=w402, y=60.0) -> (x/y=w400:dbl)
      "53" <- w400
    }
    frame 54 {
      n214 = Unbundle By Name(w413) -> ("Station Test State 54"=w408:T8)
      n215 = Equal?(x=WILT_Dryer_Test_State."Increment Cycle", y=w408) -> (x = y?=w410:bool)
      n216 = call "UTILITY E-Time.vi"("Reset"=w410) -> ("Elapsed Time (sec)"=w409:dbl)  [unwired: 8 in, 2 out]
      n217 = Divide(x=w409, y=60.0) -> (x/y=w407:dbl)
      "54" <- w407
    }
    frame 55 {
      n218 = Unbundle By Name(w420) -> ("Station Test State 55"=w415:T8)
      n219 = Equal?(x=WILT_Dryer_Test_State."Increment Cycle", y=w415) -> (x = y?=w417:bool)
      n220 = call "UTILITY E-Time.vi"("Reset"=w417) -> ("Elapsed Time (sec)"=w416:dbl)  [unwired: 8 in, 2 out]
      n221 = Divide(x=w416, y=60.0) -> (x/y=w414:dbl)
      "55" <- w414
    }
    frame 56 {
      n222 = Unbundle By Name(w427) -> ("Station Test State 56"=w422:T8)
      n223 = Equal?(x=WILT_Dryer_Test_State."Increment Cycle", y=w422) -> (x = y?=w424:bool)
      n224 = call "UTILITY E-Time.vi"("Reset"=w424) -> ("Elapsed Time (sec)"=w423:dbl)  [unwired: 8 in, 2 out]
      n225 = Divide(x=w423, y=60.0) -> (x/y=w421:dbl)
      "56" <- w421
    }
  }
  n226 = call "WILT Index Station Stats.vi"("Station Number"="Station Number", "Cool Down Period (seconds)"="Cool Down Period (seconds)", "Drying Time (Min)"="Drying Time (Min)", "Previous Run Statistics"="Previous Run Statistics", "Enable Start Retry in"="Enable Start Retry", "Error In"="Error In") -> ("Station Array Index"=w17:u32, "Station Cool Down Period (Sec)"=w14:dbl, "Station Drying Time (Min)"=w12:dbl, "Previous Cycle Time (Minutes)"=w13:dbl, "Enable Start Retry out"=w7:bool, "Error Out"=w10:errorcluster)  [unwired: 8 in]
  n227 = call "WILT Anti Flood Check.vi"("Disable Flood Check"="Disable Flood Check", "Current Station Time (Minutes)"=w5, "Error In"=w10, "Enable Start Retry"=w7, "Previous Cycle Time (Minutes)"=w13, "Station Drying Time (Min)"=w12) -> ("Error Out 2"=w8:errorcluster, "Shut Valve Off?"=w2:bool)  [unwired: 4 in]
  n228 = case shown="False" w2 {
    tunnel: ["Day/Night Cycle" WILT_Day_Night_Cycle_Enum."Day Cycle (No Water)" ("Day/Night Cycle")] -> w11
    frame False {
    }
    frame True {
    }
  }
  n229 = Index Array(array="GUI Aisle in", index="Aisle Location Index") -> (element=w29:T9)
  n230 = case shown="\"Water Injection 1 (On)\"" w31 {
    tunnel: w29 -> [w437 w447 w459 w471 w481 w491 w500 w508 w521 w531 w538 w548 w562 w571 w584 w594 w605 w613]
    tunnel: [w436 w445 w458 w470 w480 w489 w499 w509 w520 w527 w537 w546 w559 w569 w581 w592 w604 w612] -> w30
    tunnel: [w435 w446 w457 w469 w479 w493 w498 w511 w519 w528 w536 w550 w560 w573 w582 w591 w603 w611] -> w32
    tunnel: "Station Number" -> [w434 w448 w453 w472 w482 w490 w501 w507 w515 w530 w539 w547 w558 w570 w585 w593 w600 w609]
    tunnel: w8 -> [w433 w450 w456 w467 w477 w495 w503 w513 w517 w525 w534 w552 w556 w575 w579 w590 w601 w616]
    tunnel: [w432 w449 w455 w466 w476 w494 w502 w510 w516 w526 w535 w551 w555 w574 w580 w589 w602 w615] -> w33
    tunnel: "Station Test State In" -> [w431 w444 w454 w468 w478 w492 w497 w512 w518 w529 w533 w549 w561 w572 w583 w588 w606 w614]
    tunnel: w11 -> [_ _ _ w461 _ w484 _ _ _ _ _ w541 _ w564 _ _ _ w610]
    tunnel: "Injection Times" -> [_ _ _ _ w475 _ _ _ _ _ _ _ w557 _ _ _ _ _]
    tunnel: "Current Threshold" -> [_ w443 w452 _ w474 _ _ _ _ _ _ _ w554 _ w578 _ w598 _]
    tunnel: w14 -> [_ _ _ _ _ _ _ _ _ _ _ _ _ _ _ w587 _ _]
    tunnel: "Agilent Valve and Switch Locations" -> [_ w439 _ w465 _ w486 _ w506 _ w524 _ w545 _ w566 _ _ w599 _]
    tunnel: w7 -> [w430 w442 w451 w464 w473 w485 w496 w505 w514 w523 w532 w544 w553 w565 w577 w586 w597 _]
    tunnel: [w430 w442 w451 w464 w473 w485 w496 w505 w514 w523 w532 w544 w553 w565 w577 w586 w597 w608] -> w21
    tunnel: "Send Restart Every? (Sec)" -> [_ w441 _ _ _ _ _ _ _ _ _ _ _ _ _ _ _ _]
    tunnel: "Semaphore" -> [_ _ _ w460 _ w483 _ w504 _ w522 _ w540 _ w563 _ _ w596 _]
    tunnel: "Delay After Cutout (sec)" -> [_ w438 _ _ _ _ _ _ _ _ _ _ _ _ w576 _ _ _]
    tunnel: "Final Start Presses" -> [_ _ _ _ _ _ _ _ _ _ _ _ _ _ _ _ w595 _]
    tunnel: w2 -> [_ _ _ _ _ _ _ _ _ _ _ _ _ _ _ _ _ w607]
    frame "No Serial Number", Default {
      n231 = call "WILT Step 1.vi"("Station Number"=w434, "Error In"=w433, "Station Test State Cluster"=w431, "Dryer Control Input"=w437) -> ("Error Out"=w432:errorcluster, 2:"Step 1 Output"=w435:T7, 3:"Step 1 Output"=w436:T9)  [unwired: 5 in]
    }
    frame "Waiting for Dryer To Start" {
      n232 = call "WILT Step 2.vi"("Dryer Input"=w447, "Station Number in"=w448, "Send Restart Every? (Sec)"=w441, "Station Test State Cluster"=w444, "Current Threshold"=w443, "Error In"=w450, "Enable Start Retry"=w442, "Delay After Cutout (sec)"=w438, "Agilent Valve and Switch Locations"=w439) -> ("Dryer Output"=w445:T9, "Step 2 Output"=w446:T7, "Resending Sending Command"=→"Resending Sending Command":bool, "Error Out"=w449:errorcluster)  [unwired: 3 in]
    }
    frame "Drying Clothes" {
      n233 = call "WILT Step 3.vi"("Station Number in"=w453, "Error In"=w456, "Current Threshold"=w452, "Step 3 Input"=w454, "Dryer Step 3 In"=w459) -> ("Error Out"=w455:errorcluster, "Step 3 Output"=w457:T7, "Dryer Step 3 Output"=w458:T9)  [unwired: 4 in]
    }
    frame "Water Injection 1 (On)" {
      n234 = call "WILT Step 4.vi"("Dryer Step 4 In"=w471, "Day/Night Cycle"=w461, "Step 3 Input"=w468, "Error In"=w467, "Valve Status"=WILT_Water_Valve_Control."Turn Valve ON (Injection 1)", "Agilent Valve and Switch Locations"=w465, "Station Number in"=w472, "Station Group"=WILT_Room_Location."Big Room", "Semaphore"=w460) -> ("Dryer Step 4 Output"=w470:T9, "Step 3 Output"=w469:T7, "Error Out"=w466:errorcluster)  [unwired: 8 in]
    }
    frame "Water Injection 1 Timer" {
      n235 = call "WILT Injection Timer 1.vi"("Injection Times"=w475, "Station Number in"=w482, "Error In"=w477, "Current Threshold"=w474, "Step 3 Input"=w478, "Dryer Step Pause In"=w481) -> ("Error Out"=w476:errorcluster, "Step 5 Output"=w479:T7, "Dryer Step Pause Output"=w480:T9)  [unwired: 3 in]
    }
    frame "Water Injection 1 (Off)" {
      n236 = call "WILT Step 4.vi"("Dryer Step 4 In"=w491, "Day/Night Cycle"=w484, "Step 3 Input"=w492, "Error In"=w495, "Valve Status"=WILT_Water_Valve_Control."Turn Valve OFF (Injection 1)", "Agilent Valve and Switch Locations"=w486, "Station Number in"=w490, "Station Group"=WILT_Room_Location."Big Room", "Semaphore"=w483) -> ("Dryer Step 4 Output"=w489:T9, "Step 3 Output"=w493:T7, "Error Out"=w494:errorcluster)  [unwired: 8 in]
    }
    frame "Pause Dryer" {
      # "The Pause Dryer Step is intermittant to the \nSend Start Stop CMD"
      n237 = call "WILT Step Pause Dryer.vi"("Station Number in"=w501, "Error In"=w503, "Step 3 Input"=w497, "Dryer Step Pause In"=w500) -> ("Error Out"=w502:errorcluster, "Step 5 Output"=w498:T7, "Dryer Step Pause Output"=w499:T9)  [unwired: 5 in]
    }
    frame "Sending Start Stop CMD" {
      n238 = call "WILT Send Start Stop CMD.vi"("Dryer Step 4 In"=w508, "Step 3 Input"=w512, "Error In"=w513, "Station Number in"=w507, "Agilent Valve and Switch Locations"=w506, "Semaphore"=w504) -> ("Dryer Step 4 Output"=w509:T9, "Step 3 Output"=w511:T7, "Error Out"=w510:errorcluster)  [unwired: 11 in]
    }
    frame "Pause Dryer 2" {
      n239 = call "WILT Step 5.vi"("Station Number in"=w515, "Error In"=w517, "Step 3 Input"=w518, "Dryer Step 5 In"=w521) -> ("Error Out"=w516:errorcluster, "Step 5 Output"=w519:T7, "Dryer Step 5 Output"=w520:T9)  [unwired: 5 in]
    }
    frame "Sending Start Stop CMD 2" {
      n240 = call "WILT Send Start Stop CMD.vi"("Dryer Step 4 In"=w531, "Step 3 Input"=w529, "Error In"=w525, "Station Number in"=w530, "Agilent Valve and Switch Locations"=w524, "Semaphore"=w522) -> ("Dryer Step 4 Output"=w527:T9, "Step 3 Output"=w528:T7, "Error Out"=w526:errorcluster)  [unwired: 11 in]
    }
    frame "Drying Clothes 2" {
      n241 = call "WILT Step 6.vi"("Station Number in"=w539, "Error In"=w534, "Step 3 Input"=w533, "Dryer Step 5 In"=w538) -> ("Error Out"=w535:errorcluster, "Step 5 Output"=w536:T7, "Dryer Step 5 Output"=w537:T9)  [unwired: 5 in]
    }
    frame "Water Injection 2 (On)" {
      n242 = call "WILT Step 4.vi"("Dryer Step 4 In"=w548, "Day/Night Cycle"=w541, "Step 3 Input"=w549, "Error In"=w552, "Valve Status"=WILT_Water_Valve_Control."Turn Valve ON (Injection 2)", "Agilent Valve and Switch Locations"=w545, "Station Number in"=w547, "Station Group"=WILT_Room_Location."Big Room", "Semaphore"=w540) -> ("Dryer Step 4 Output"=w546:T9, "Step 3 Output"=w550:T7, "Error Out"=w551:errorcluster)  [unwired: 8 in]
    }
    frame "Water Injection 2 Timer" {
      n243 = call "WILT Injection Timer 2.vi"("Injection Times"=w557, "Station Number in"=w558, "Error In"=w556, "Current Threshold"=w554, "Step 3 Input"=w561, "Dryer Step Pause In"=w562) -> ("Error Out"=w555:errorcluster, "Step 5 Output"=w560:T7, "Dryer Step Pause Output"=w559:T9)  [unwired: 3 in]
    }
    frame "Water Injection 2 (Off)" {
      n244 = call "WILT Step 4.vi"("Dryer Step 4 In"=w571, "Day/Night Cycle"=w564, "Step 3 Input"=w572, "Error In"=w575, "Valve Status"=WILT_Water_Valve_Control."Turn Valve OFF (Injection 2)", "Agilent Valve and Switch Locations"=w566, "Station Number in"=w570, "Station Group"=WILT_Room_Location."Big Room", "Semaphore"=w563) -> ("Dryer Step 4 Output"=w569:T9, "Step 3 Output"=w573:T7, "Error Out"=w574:errorcluster)  [unwired: 8 in]
    }
    frame "Drying Clothes 3" {
      n245 = call "WILT Step Drying Clothes 3.vi"("Delay After Cutout (sec)"=w576, "Station Number in"=w585, "Error In"=w579, "Current Threshold"=w578, "Station Test State Cluster"=w583, "Dryer Input"=w584) -> ("Error Out"=w580:errorcluster, "Step 2 Output"=w582:T7, "Dryer Output"=w581:T9)  [unwired: 3 in]
    }
    frame "Cooling Down" {
      n246 = call "WILT Step Cooling Down.vi"("Cool Down Period (seconds)"=w587, "Station Number in"=w593, "Error In"=w590, "Step 3 Input"=w588, "Dryer Step 5 In"=w594) -> ("Error Out"=w589:errorcluster, "Step 5 Output"=w591:T7, "Dryer Step 5 Output"=w592:T9)  [unwired: 4 in]
    }
    frame "Sending Start Stop CMD 3" {
      n247 = call "WILT Send Start Stop CMD.vi"("Dryer Step 4 In"=w605, "Step 3 Input"=w606, "Final Start Presses"=w595, "Error In"=w601, "Current Threshold"=w598, "Station Number in"=w600, "Agilent Valve and Switch Locations"=w599, "Semaphore"=w596) -> ("Dryer Step 4 Output"=w604:T9, "Step 3 Output"=w603:T7, "Error Out"=w602:errorcluster)  [unwired: 9 in]
    }
    frame "Increment Cycle" {
      n248 = call "WILT Increment Cycle.vi"("Station Number in"=w609, "Short Cycle?"=w607, "Day/Night Cycle"=w610, "Error In"=w616, "Station Test State In"=w614, "Dryer Step 5 In"=w613) -> ("Error Out"=w615:errorcluster, "Enable Start Retry"=w608:bool, "Test Station Out"=w611:T7, "Dryer Step 5 Output"=w612:T9)  [unwired: 2 in]
    }
  }
  "Error Out" <- w33
  "Test Station Out" <- w32
  n249 = Replace Array Subset(array="GUI Aisle in", new element=w30, index="Aisle Location Index") -> (→"GUI Aisle 1":T9[])
  n250 = Replace Array Subset(array="Enable Start Retry", new element=w21, index=w17) -> (→"Enable Start Retry Out":bool[])
